vi "Transform3d_Create_Default.vi"() -> (3 "Transform3d":T1={"TRANSLATION3D"={"X"=0.0, "Y"=0.0, "Z"=0.0}, "ROTATION3D"={"Q_quaternion"={"R"=1.0, "V"=[0.0, 0.0, 0.0]}}} {"TRANSLATION3D"."Z" format="%14.3f"; "TRANSLATION3D"."Y" format="%14.3f"; "TRANSLATION3D"."X" format="%14.3f"})   [LabVIEW 2019, in "Trajectory_Library.lvlib"]
doc: "Constructs a transform with the given translation and rotation components.\n\nParameters:\n - translation -Translational component of the transform.\n - rotation - Rotational component of the transform.\n\nResult:\n - transform - TRANSFORM data structure"
uses:
  Trajectory_Library.lvlib
  TRANSFORM3D.ctl
  TRANSLATION3D.ctl
  ROTATION3D.ctl
  QUATERNION.ctl
  Quaternion_New_Default.vi
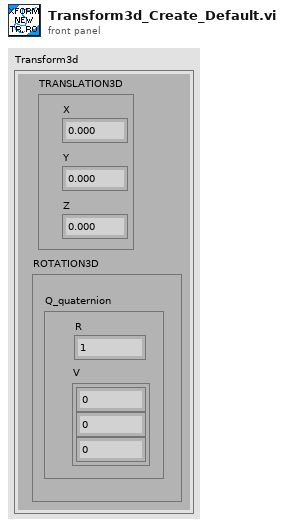
[diagram p1: front panel]
types:
  T1 = typedef "Trajectory_Library.lvlib/TRANSFORM3D.ctl" = cluster{"TRANSLATION3D":T2, "ROTATION3D":T3}
  T2 = typedef "Trajectory_Library.lvlib/TRANSLATION3D.ctl" = cluster{"X":dbl, "Y":dbl, "Z":dbl}
  T3 = typedef "Trajectory_Library.lvlib/ROTATION3D.ctl" = cluster{"Q_quaternion":T4}
  T4 = typedef "Trajectory_Library.lvlib/QUATERNION.ctl" = cluster{"R":dbl, "V":dbl[]}
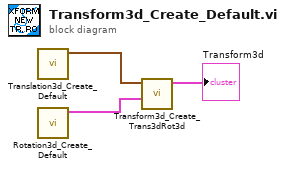
[diagram p0: block diagram]
diagram:
  n1 = call "Translation3d_Create_Default.vi"() -> ("TRANSLATION3D"=w2:T2)  [unwired: 11 in]
  n2 = call "Rotation3d_Create_Default.vi"() -> ("ROTATION3D"=w1:T3)  [unwired: 11 in]
  n3 = call "Transform3d_Create_Trans3dRot3d.vi"("Rotation3d"=w1, "Translation3d"=w2) -> ("Transform3d"=→"Transform3d":T1)  [unwired: 9 in]
